vi "Add Tool Offset.vi"(11 "XYZTheta":dbl[](array[numeric])) -> (3 "Array":dbl[](array[numeric]))   [LabVIEW 2019, in "Pick and Place.lvclass"]
uses:
  Pick and Place.lvclass
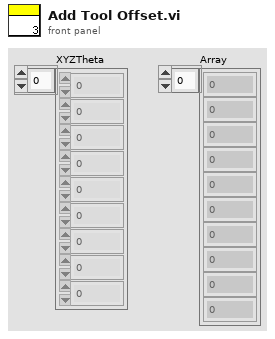
[diagram p1: front panel]
types:
  T1 = typedef "File Paths.ctl" = cluster{"Glue Pattern Folder":path, "Carrier Tray Folder":path, "Pick Up Tool Fixture Folder":path, "Components Folder":path, "Bellows Tool Offset.txt":path, "Pick Up Tool Offset.txt":path, "Dispense Tip Offset.txt":path, "Log Files":path}
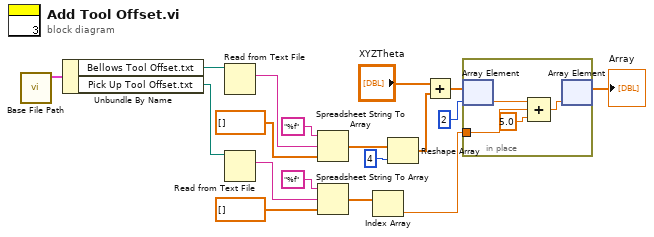
[diagram p0: block diagram]
diagram:
  n1 = call "Base File Path.vi"() -> ("Paths Out"=w10:T1)  [unwired: 11 in]
  n2 = Unbundle By Name(w10) -> ("Bellows Tool Offset.txt"=w11:path, "Pick Up Tool Offset.txt"=w3:path)
  n3 = Read from Text File(file (use dialog)=w11) -> (text=w12:string)  [unwired: 3 in, 3 out]
  n4 = Read from Text File(file (use dialog)=w3) -> (text=w6:string)  [unwired: 3 in, 3 out]
  n5 = Spreadsheet String To Array(format string="%f", spreadsheet string=w12, array type (2D Dbl)=dbl[] []) -> (array=w15:dbl[])  [unwired: 1 in]
  n6 = Spreadsheet String To Array(format string="%f", spreadsheet string=w6, array type (2D Dbl)=dbl[] []) -> (array=w2:dbl[])  [unwired: 1 in]
  n7 = Index Array(array=w2) -> (element=w1:dbl)  [unwired: 1 in]
  n8 = Reshape Array(w15, 4 ("dimension size")) -> (w17:dbl[])
  n9 = Add(x="XYZTheta", y=w17) -> (x+y=w9:dbl[])
  n10 = in-place {
    in-place-border: w1 -> [w21]
    n11 = in-place-array #1(w9, 2) -> (w22:dbl)
    n12 = Compound Arithmetic op=ADD(w22, w21, 5.0 ("x")) -> (w19:dbl)
    n13 = in-place-array #1(w19) -> (→"Array":dbl[])  [unwired: 1 out]
  }
